vi "Set Up Dialog - Gas Pressure.vi"() -> ()   [LabVIEW 2012]
panel:
  out "Calibration Instructions":string="1. Connect the sensor to your myDAQ as shown in the diagram above.\n\n2.  Ensure the manometer on the blood pressure cuff is at 0mmHg. Record voltage for SP1\n\n3. Using the manometer apply 200mmHg, ensure the signal is steady and record voltage for set for SP2."
  # "iWorx - Gas Pressure - Set Up"
  # "Gas Pressure Sensor GPSN-100"
  # "iWorx"
  # "Sensor"
  # "GPSN - 100"
  # "myDAQ"
  # "Computer"
  # "Adaptor"
  # "Connection Diagram"
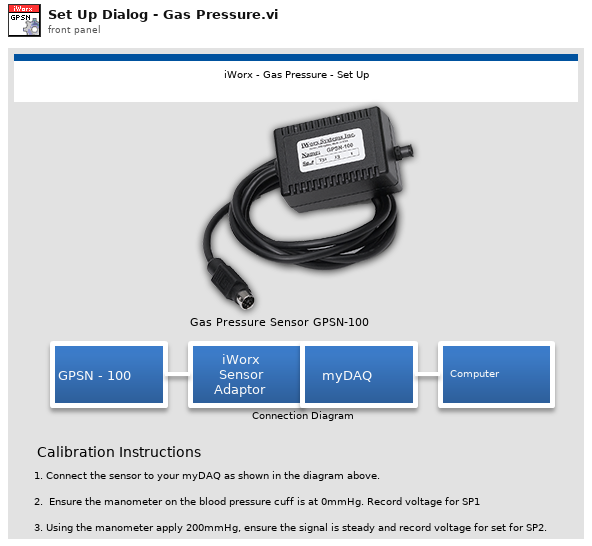
[diagram p1: front panel]
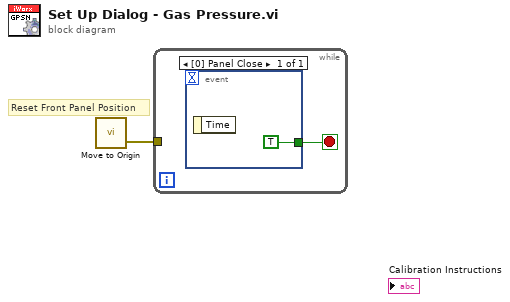
[diagram p0: block diagram]
diagram:
  # "Reset Front Panel Position"
  n1 = call "Move to Origin.vi"() -> ("Error Out"=w1:errorcluster)  [unwired: 3 in]
  n2 = while {
    tunnel: w1 -> [_]
    stop <- w2 stop-if-true
    n3 = event shown="[0] Panel Close" {
      selector: _ -> [_]
      dyn-events: _ -> [_]
      timeout: _ -> [_]
      tunnel: [TRUE] -> w2
      event Panel Close {
        n4 = event-data() -> ()  [unwired: 1 in, 1 out]
      }
    }
  }
